vi "Strip Parent Folder.vi"(8 "Root RT Path In":string, 9 "Modified RT Path In":string) -> (2 "String Path Out":string)   [LabVIEW 2023]
panel:
  out "replaced substring":string
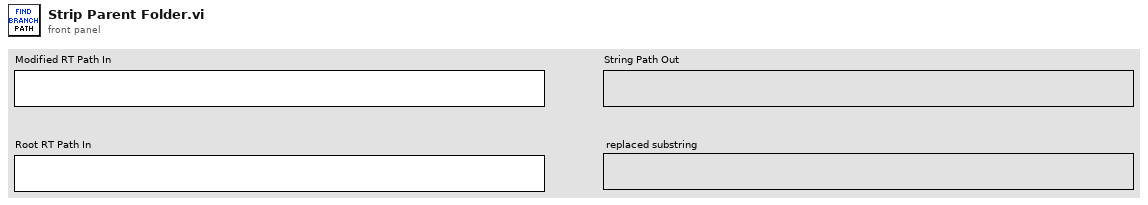
[diagram p1: front panel]
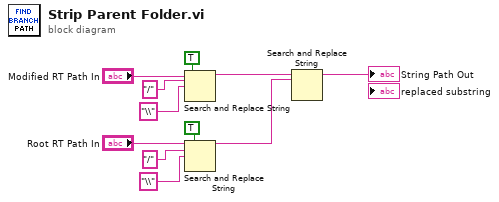
[diagram p0: block diagram]
diagram:
  n1 = Search and Replace String(replace all?=TRUE ("replace all? (F)"), input string="Modified RT Path In", search string="/", replace string="\\" ("replace string (\"\")")) -> (result string=w3:string)  [unwired: 4 in, 3 out]
  n2 = Search and Replace String(replace all?=TRUE ("replace all? (F)"), input string="Root RT Path In", search string="/", replace string="\\" ("replace string (\"\")")) -> (result string=w2:string)  [unwired: 4 in, 3 out]
  n3 = Search and Replace String(input string=w3, search string=w2) -> (result string=→"String Path Out":string)  [unwired: 6 in, 3 out]
